vi "Test Move Cursor into ROI 1.vi"(11 "Test Case In":refnum<class "test Move Cursor into ROI.lvclass">) -> (0 "error out":errorcluster, 3 "Test Case Out":refnum<class "test Move Cursor into ROI.lvclass">)   [LabVIEW 2023, in "test Move Cursor into ROI.lvclass"]
uses:
  test Move Cursor into ROI.lvclass
  C:/Program Files/National Instruments/LabVIEW 2023/vi.lib/Astemes/LUnit/Test Case.lvclass
  <vilib>/Utility/miscctls.llb/LVPointDoubleTypeDef.ctl
  source/Base Graph/Base Graph.lvclass/Base Graph.ctl
  <vilib>/Astemes/LUnit/Test Case.lvclass/Test Case.ctl
  <vilib>/Astemes/LUnit/Append Fail Result.vi
  <vilib>/Astemes/LUnit/Append Pass Result.vi
  <vilib>/Astemes/LUnit/Run In UI.vi
  <vilib>/Utility/error.llb/Clear Errors.vi
  test Move Cursor into ROI.lvclass/test Move Cursor into ROI.ctl
  source/Base Graph/Base Graph.lvclass
  <vilib>/Astemes/LUnit/Test Case.lvclass
panel:
  out "Intensity Graph":dbl[][](graph)
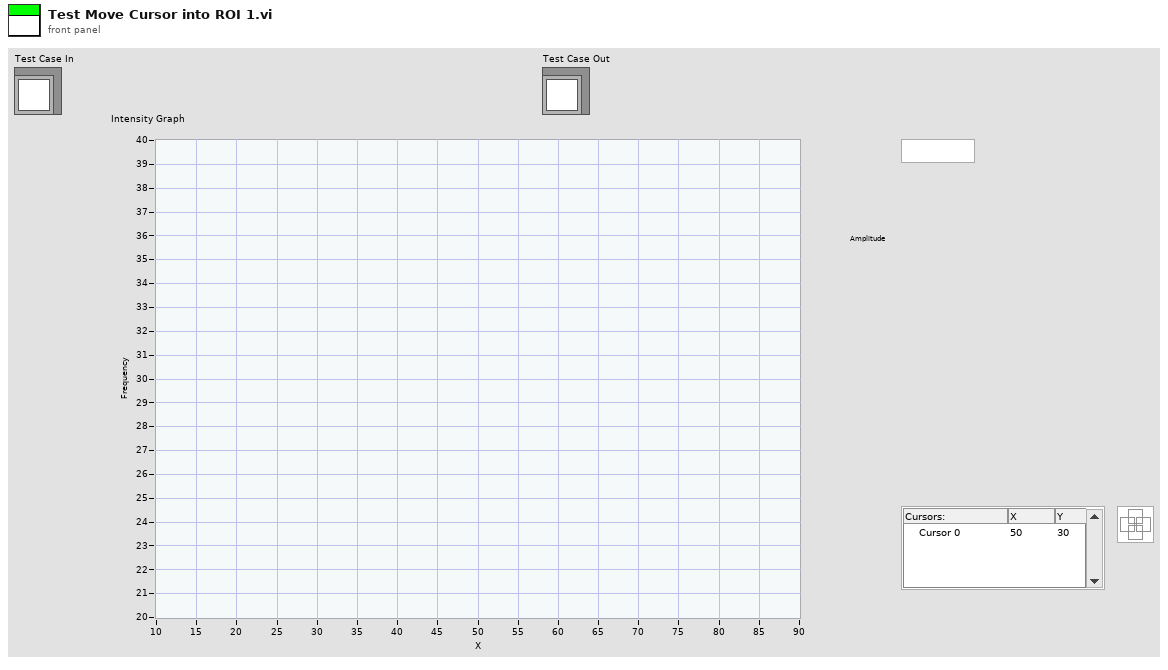
[diagram p1: front panel]
types:
  T1 = typedef "LVPointDoubleTypeDef.ctl" = cluster{"X":dbl, "Y":dbl}
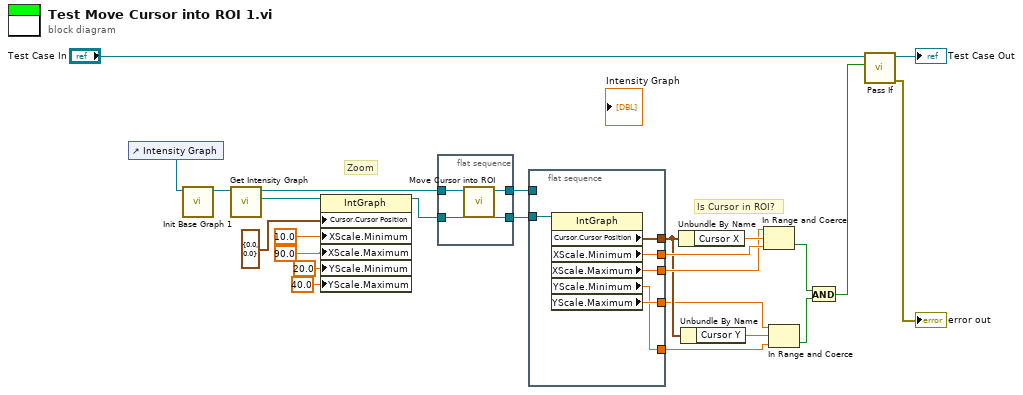
[diagram p0: block diagram]
diagram:
  # "Is Cursor in ROI?"
  # "Zoom"
  n1 = control-ref of="Intensity Graph"() -> (w25:refnum<vi>)
  n2 = call "Init Base Graph 1.vi"("IntensityGraph in"=w25) -> ("Base Graph out"=w24:refnum<class "Base Graph.lvclass">)  [unwired: 10 in]
  n3 = call "Get Intensity Graph.vi"("Base Graph in"=w24) -> ("Intensity Graph"=w22:refnum<vi>, "Base Graph out"=w23:refnum<class "Base Graph.lvclass">)  [unwired: 9 in]
  n4 = property class="IntGraph"(reference=w22, "Cursor.Cursor Position"=T1 {"X"=0.0, "Y"=0.0}, "XScale.Minimum"=10.0 ("X Scale.Range:Minimum"), "XScale.Maximum"=90.0 ("X Scale.Range:Maximum"), "YScale.Minimum"=20.0 ("Y Scale.Range:Minimum"), "YScale.Maximum"=40.0 ("Y Scale.Range:Maximum")) -> (reference out=w2:refnum<vi>)  [unwired: 1 in, 1 out]
  n5 = flat-sequence {
    tunnel: w23 -> [w28]
    tunnel: [w27] -> w13
    tunnel: w2 -> [w26]
    tunnel: [w26] -> w1
    frame #0 {
      n6 = call "Move Cursor into ROI.vi"("Base Graph in"=w28) -> ("Base Graph out"=w27:refnum<class "Base Graph.lvclass">)  [unwired: 10 in]
    }
  }
  n7 = flat-sequence {
    tunnel: w1 -> [w34]
    tunnel: w13 -> [_]
    tunnel: [w33] -> w9
    tunnel: [w32] -> w11
    tunnel: [w31] -> w10
    tunnel: [w30] -> w7
    tunnel: [w29] -> w6
    frame #0 {
      n8 = property class="IntGraph"(reference=w34) -> ("Cursor.Cursor Position"=w33:T1, "XScale.Minimum"=w32:dbl, "XScale.Maximum"=w31:dbl, "YScale.Minimum"=w29:dbl, "YScale.Maximum"=w30:dbl)  [unwired: 1 in, 2 out]
    }
  }
  n9 = Unbundle By Name(w9) -> ("Cursor X"=w12:dbl)
  n10 = Unbundle By Name(w9) -> ("Cursor Y"=w8:dbl)
  n11 = In Range and Coerce(upper limit=w10, x=w12, lower limit=w11) -> (In Range?=w4:bool)  [unwired: 1 out]
  n12 = In Range and Coerce(upper limit=w7, x=w8, lower limit=w6) -> (In Range?=w5:bool)  [unwired: 1 out]
  n13 = And(x=w4, y=w5) -> (x .and. y?=w3:bool)
  n14 = call <vilib>:"Pass If.vi"("Pass?"=w3, "LUnit Test Case In"="Test Case In") -> ("error out"=→"error out":errorcluster, "LUnit Test Case Out"=→"Test Case Out":refnum<class "test Move Cursor into ROI.lvclass">)  [unwired: 8 in]
